vi "Dequeue.vi"(8 "Error In":errorcluster, 9 "timeout in ms (-1)":i32=-1) -> (0 "error out":errorcluster, 1 "State":T2=enum."DoSomething", 2 "Data out":T1={"State"=enum."DoSomething", "Payload"=variant, "WaitOnReply"=FALSE, "ReplyNotif"=refnum})   [LabVIEW 2018, in "Controller.lvlib"]
uses:
  Controller.lvlib
  States_Module.ctl
  MessageData.ctl
  States_FGVQ.ctl
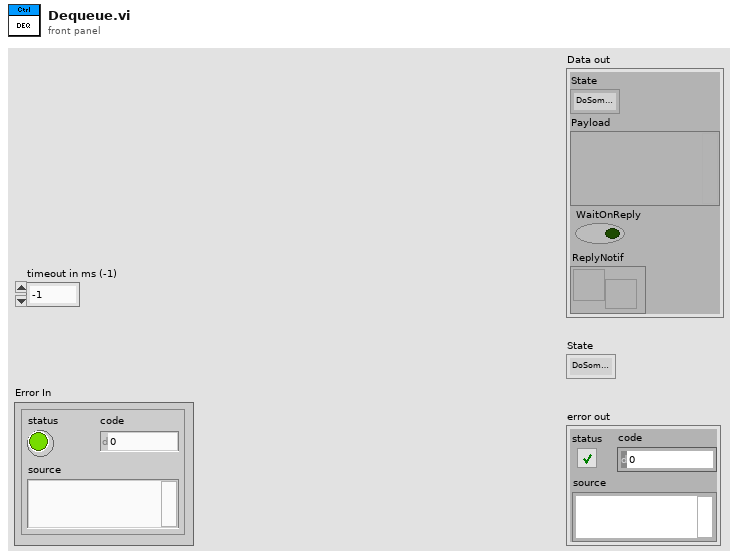
[diagram p1: front panel]
types:
  T1 = typedef "Controller.lvlib/MessageData.ctl" = cluster{"State":T2, "Payload":variant, "WaitOnReply":bool, "ReplyNotif":refnum<notifier>}
  T2 = typedef "Controller.lvlib/States_Module.ctl" = enum16{"Array2Cluster", "ProcessXLS", "DoSomething", "Shutdown", "Initialize", "RequestOracleReport"}
  T3 = typedef "Controller.lvlib/States_FGVQ.ctl" = enum16{"Get", "Shutdown", "Initialize"}
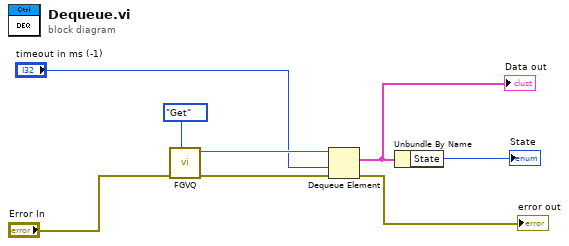
[diagram p0: block diagram]
diagram:
  n1 = call "FGVQ.vi"("State"=States_FGVQ."Get", "Error In"="Error In") -> ("Error Out"=w7:errorcluster, "queue out"=w6:refnum<queue>)  [unwired: 8 in]
  n2 = Dequeue Element(queue=w6, timeout in ms (-1)="timeout in ms (-1)", error in (no error)=w7) -> (element=w5:T1, error out=→"error out":errorcluster)  [unwired: 2 out]
  "Data out" <- w5
  n3 = Unbundle By Name(w5) -> ("State"=→"State":T2)
